vi "pAnalyzeSequence.vi"(11 "Array 3":string[][](array[string])) -> (3 "Sequence":T1)   [LabVIEW 2013]
uses:
  Controls/SequenceCluster.ctl
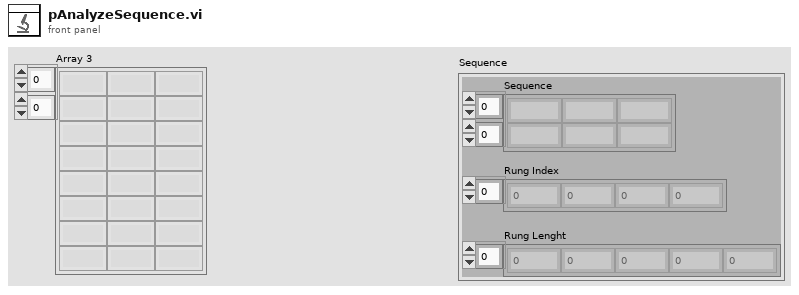
[diagram p1: front panel]
types:
  T1 = typedef "SequenceCluster.ctl" = cluster{"Sequence":string[][], "Rung Index":i32[], "Rung Lenght":i32[]}
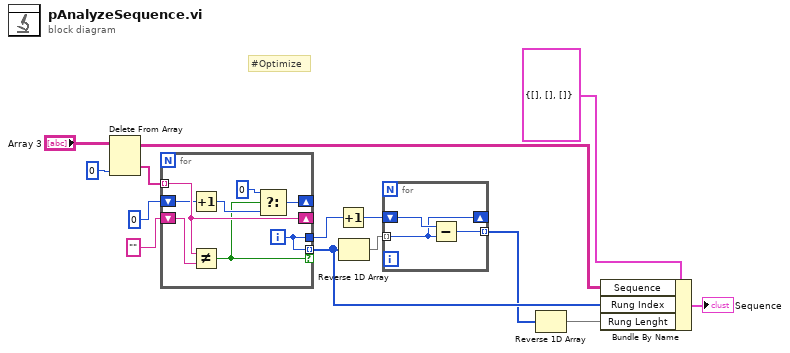
[diagram p0: block diagram]
diagram:
  # "#Optimize"
  n1 = Delete From Array(array="Array 3", index (col)=0 ("disabled index (col)")) -> (deleted portion=w14:string[], array with subset deleted=w8:string[][])  [unwired: 2 in]
  n2 = for {
    tunnel: w14 -> [w21] mode=indexing
    shift-right: [w21] -> _
    shift-left: "" ("String") -> [w22]
    tunnel: [w15] -> w4 mode=indexing if=w16
    shift-right: [w19] -> _
    shift-left: 0 -> [w18]
    tunnel: [w15] -> w6
    i -> [w15]
    n3 = Increment(x=w18) -> (x+1=w17:i32)
    n4 = Not Equal?(x=w21, y=w22) -> (x != y?=w16:bool)
    n5 = Select(t=0, s=w16, f=w17) -> (s? t:f=w19:i32)
  }
  n6 = Increment(x=w6) -> (x+1=w5:i32)
  n7 = Reverse 1D Array(array=w4) -> (reversed array=w2:i32[])
  n8 = for {
    tunnel: w2 -> [w23] mode=indexing
    shift-right: [w23] -> _
    shift-left: w5 -> [w25]
    tunnel: [w24] -> w3 mode=indexing
    n9 = Subtract(x=w25, y=w23) -> (x-y=w24:i32)
  }
  n10 = Reverse 1D Array(array=w3) -> (reversed array=w1:i32[])
  n11 = Bundle By Name(cluster=T1 {"Sequence"=[], "Rung Index"=[], "Rung Lenght"=[]} ("Sequence"), "Sequence"=w8, "Rung Index"=w4, "Rung Lenght"=w1) -> (→"Sequence":T1)
